vi "Modify Package BuildSpec Version Example.vi"() -> ()   [LabVIEW 2018]
uses:
  <vilib>/AppBuilder/AB_API_Simple/Build Specification Version.ctl
  Package Build Specification API (2018)/NIPKG BuildSpec API.lvlib
  <vilib>/AppBuilder/AB_API_Simple/NI_App_Builder_API.lvlib
  <vilib>/AppBuilder/AB_API_Simple/Get Build Specification Version (path).vi
  <vilib>/AppBuilder/AB_API_Simple/Set Build Specification Version (path).vi
panel:
  out "version updated?":bool
  in  "Package build spec name":string
  out "Build Spec Version (Initial)":T1
  out "Build Spec Version (Final)":T1
  in  "LabVIEW project filepath":path
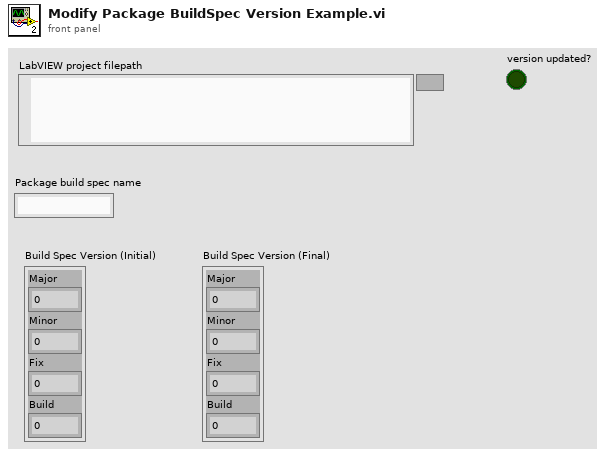
[diagram p1: front panel]
types:
  T1 = typedef "NI_App_Builder_API.lvlib/Build Specification Version.ctl" = cluster{"Major":u16, "Minor":u16, "Fix":u16, "Build":u16}
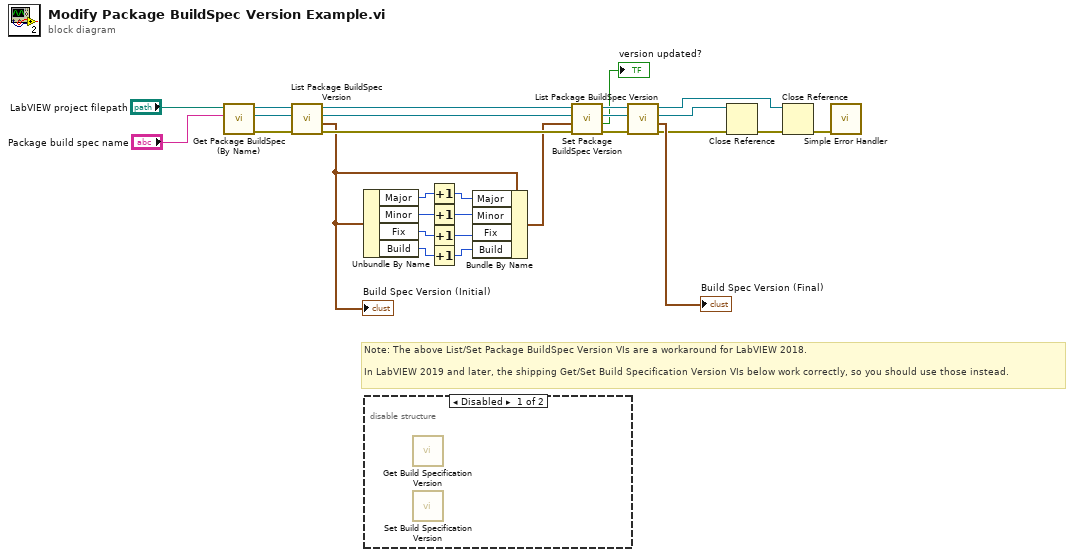
[diagram p0: block diagram]
diagram:
  # "Note: The above List/Set Package BuildSpec Version VIs are a workaround for LabVIEW 2018.\n\nIn LabVIEW 2019 and later, the shipping Get/Set Build Specification Version VIs below work correctly, so you should use those instead."
  n1 = call "Get Package BuildSpec (By Name).vi"("package build spec name"="Package build spec name", "LabVIEW project filepath"="LabVIEW project filepath") -> ("error out"=w3:errorcluster, "package build spec ref out"=w4:refnum<vi>, "project ref out"=w5:refnum<vi>)  [unwired: 7 in]
  n2 = call "List Package BuildSpec Version.vi"("error in (no error)"=w3, "package buildspec ref in"=w4, "project ref in"=w5) -> ("error out"=w27:errorcluster, "Build Specification Version"=w13:T1, "package buildspec ref out"=w24:refnum<vi>, "project ref out"=w25:refnum<vi>)  [unwired: 5 in]
  "Build Spec Version (Initial)" <- w13
  n3 = Unbundle By Name(w13) -> ("Major"=w14:u16, "Minor"=w20:u16, "Fix"=w18:u16, "Build"=w16:u16)
  n4 = disable-structure shown="Disabled" {
    frame Disabled {
      n5 = call-poly <vilib>:"Get Build Specification Version.vi"() -> ()  [unwired: 10 in, 2 out]
      n6 = call-poly <vilib>:"Set Build Specification Version.vi"() -> ()  [unwired: 11 in, 1 out]
    }
    frame Enabled {
    }
  }
  n7 = Increment(x=w14) -> (x+1=w21:u16)
  n8 = Increment(x=w20) -> (x+1=w19:u16)
  n9 = Increment(x=w18) -> (x+1=w17:u16)
  n10 = Increment(x=w16) -> (x+1=w15:u16)
  n11 = Bundle By Name(cluster=w13, "Major"=w21, "Minor"=w19, "Fix"=w17, "Build"=w15) -> (w12:T1)
  n12 = call "Set Package BuildSpec Version.vi"("error in (no error)"=w27, "Build Specification Version"=w12, "package buildspec ref in"=w24, "project ref in"=w25) -> ("error out"=w26:errorcluster, "version updated?"=→"version updated?":bool, "package buildspec ref out"=w22:refnum<vi>, "project ref out"=w23:refnum<vi>)  [unwired: 4 in]
  n13 = call "List Package BuildSpec Version.vi"("error in (no error)"=w26, "package buildspec ref in"=w22, "project ref in"=w23) -> ("error out"=w8:errorcluster, "Build Specification Version"=→"Build Spec Version (Final)":T1, "package buildspec ref out"=w9:refnum<vi>, "project ref out"=w10:refnum<vi>)  [unwired: 5 in]
  n14 = Close Reference(reference=w9, error in (no error)=w8) -> (error out=w28:errorcluster)
  n15 = Close Reference(reference=w10, error in (no error)=w28) -> (error out=w7:errorcluster)
  n16 = call <vilib>:"Simple Error Handler.vi"("error in (no error)"=w7) -> ()  [unwired: 4 in, 5 out]
